vi "Actor Core.vi"(8 "error in (no error)":errorcluster, 11 "MC Screen.lvlib:MC Screen.lvclass":refnum<class "Grid Screen.lvclass">) -> (0 "error out":errorcluster, 3 "Actor out":refnum<class "Actor.lvclass">)   [LabVIEW 2024, in "Grid Screen.lvlib" / "Grid Screen.lvclass"]
uses:
  Grid Screen.lvclass
  <vilib>/ActorFramework/Actor/Actor.lvclass
  <vilib>/Utility/miscctls.llb/LVRectTypeDef.ctl
  Grid Screen.lvclass/Grid Screen.ctl
  <vilib>/ActorFramework/Actor/Actor.lvclass/Actor.ctl
  <vilib>/ActorFramework/Message Enqueuer/Message Enqueuer.lvclass/Message Enqueuer.ctl
  Grid Screen Messages/Button Pressed Msg/Button Pressed Msg.lvclass/Button Pressed Msg.ctl
  <vilib>/ActorFramework/Message Enqueuer/Init from Existing Queue.vi
  <vilib>/ActorFramework/Message Enqueuer/Enqueue.vi
  Grid Screen Messages/Button Pressed Msg/Button Pressed Msg.lvclass
  <vilib>/ActorFramework/Stop Msg/Stop Msg.lvclass
  <vilib>/ActorFramework/Message Priority Queue/Priority Enqueue.vi
  <vilib>/ActorFramework/Message Enqueuer/Message Enqueuer.lvclass
panel:
  out "Cat 1":string="CATEGORY 1"
  out "Cat 2":string="CATEGORY 2"
  out "Cat 3":string="CATEGORY 3"
  out "Cat 4":string="CATEGORY 4"
  out "Cat 5":string="CATEGORY 5"
  out "A1":bool
  out "A2":bool
  out "A3":bool
  out "A4":bool
  out "A5":bool
  out "B1":bool
  out "B2":bool
  out "B3":bool
  out "B4":bool
  out "B5":bool
  out "C1":bool
  out "C2":bool
  out "C3":bool
  out "C4":bool
  out "C5":bool
  out "D1":bool
  out "D2":bool
  out "D3":bool
  out "D4":bool
  out "D5":bool
  out "E1":bool
  out "E2":bool
  out "E3":bool
  out "E4":bool
  out "E5":bool
  in  "Stop":bool
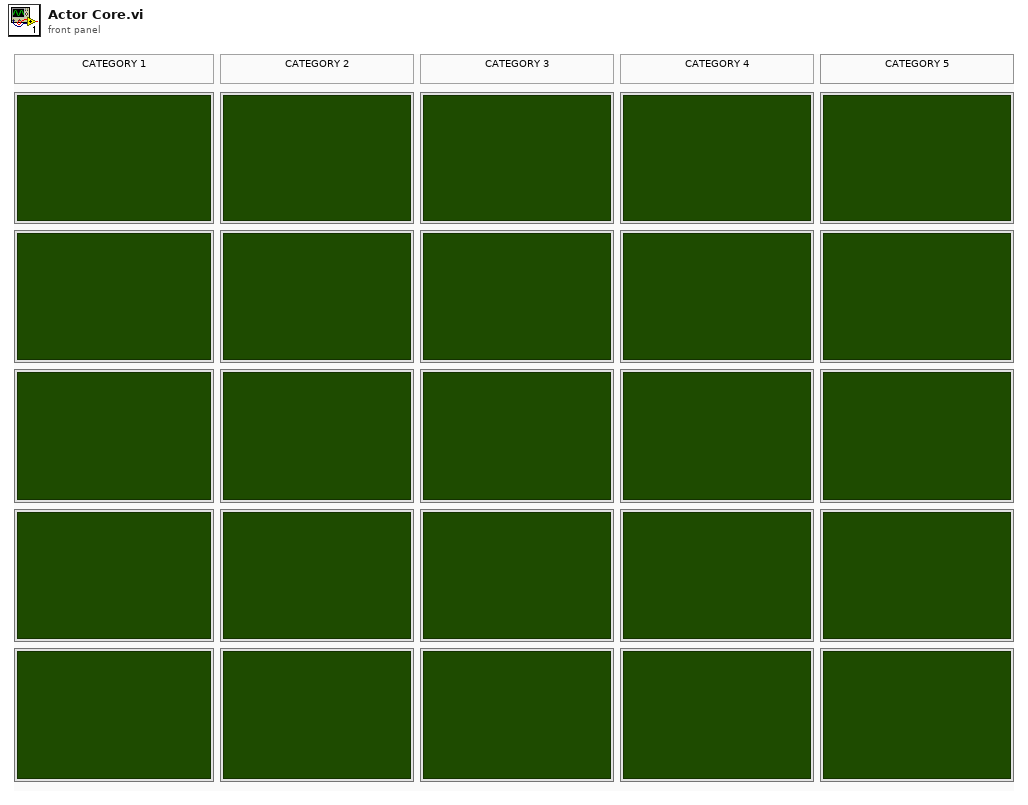
[diagram p1: front panel]
types:
  T1 = enum16{"Sticks Top/Left", "Sticks Bottom/Right", "Proportional"}
  T2 = typedef "LVRectTypeDef.ctl" = cluster{"Left":i16, "Top":i16, "Right":i16, "Bottom":i16}
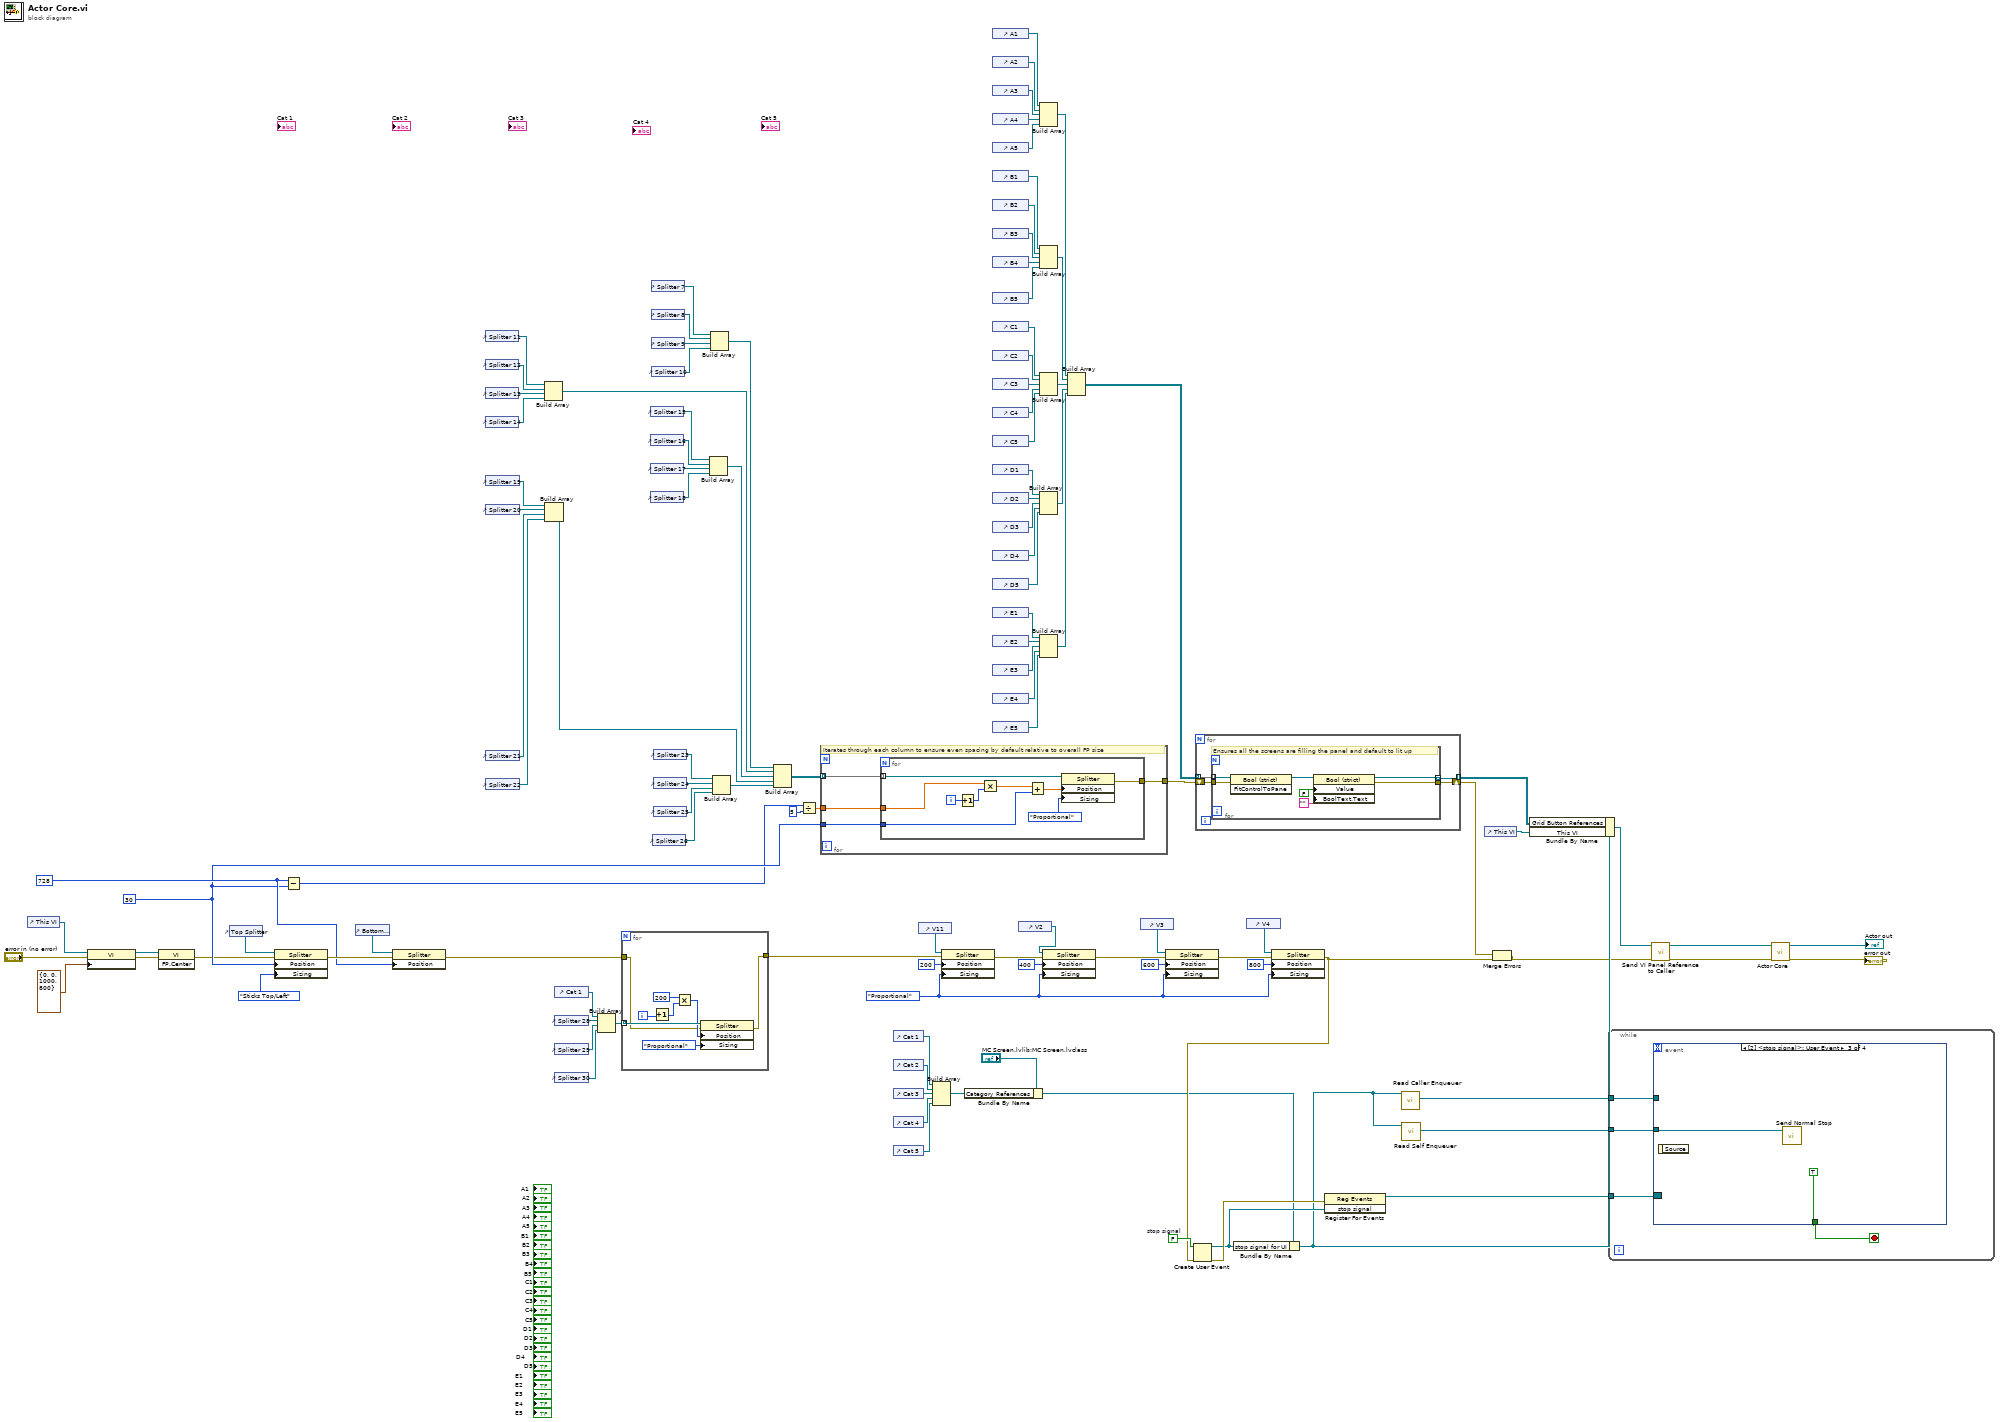
[diagram p0: block diagram]
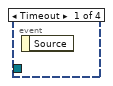
[diagram p2: hidden frame]
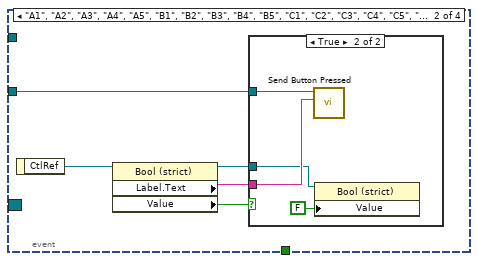
[diagram p3: hidden frame]
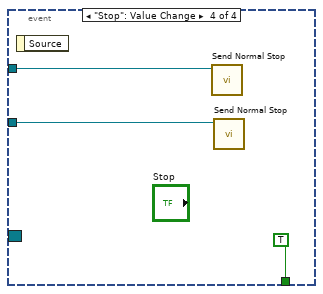
[diagram p5: hidden frame]
diagram:
  w63 = FALSE  # stop signal
  w105 = T1."Proportional" ("Sizing")
  w74 = 728 ("Splitter Position")
  w73 = 30 ("Splitter Position")
  n1 = control-ref of="This VI"() -> (w46:refnum<vi>)
  n2 = property class="VI"(reference=w46, error in="error in (no error)", "Front Panel.WinBounds"=T2 {"Left"=0, "Top"=0, "Right"=1000, "Bottom"=800} ("Front Panel Window:Window Bounds")) -> (reference out=w60:refnum<vi>, error out=w61:errorcluster)
  n3 = invoke class="VI" method="FP.Center"(reference=w60, error in=w61) -> (error out=w54:errorcluster)  [unwired: 1 in, 2 out]
  n4 = control-ref of="Top Splitter"() -> (w116:refnum<vi>)
  n5 = property class="Splitter"(reference=w116, error in=w54, "Position"=w73, "Sizing"=T1."Sticks Top/Left") -> (error out=w114:errorcluster)  [unwired: 1 out]
  n6 = Subtract(x=w74, y=w73) -> (x-y=w72:i32)
  n7 = control-ref of="Bottom Splitter"() -> (w115:refnum<vi>)
  n8 = property class="Splitter"(reference=w115, error in=w114, "Position"=w74) -> (error out=w53:errorcluster)  [unwired: 1 out]
  n9 = control-ref of="Splitter 11"() -> (w96:refnum<vi>)
  n10 = control-ref of="Splitter 12"() -> (w95:refnum<vi>)
  n11 = control-ref of="Splitter 13"() -> (w82:refnum<vi>)
  n12 = control-ref of="Splitter 14"() -> (w81:refnum<vi>)
  n13 = control-ref of="Splitter 19"() -> (w84:refnum<vi>)
  n14 = control-ref of="Splitter 20"() -> (w91:refnum<vi>)
  n15 = control-ref of="Splitter 21"() -> (w90:refnum<vi>)
  n16 = control-ref of="Splitter 22"() -> (w89:refnum<vi>)
  n17 = Build Array(w96, w95, w82, w81) -> (w79:refnum<vi>[])
  n18 = Build Array(w84, w91, w90, w89) -> (w77:refnum<vi>[])
  n19 = control-ref of="Cat 1"() -> (w56:refnum<vi>)
  n20 = control-ref of="Splitter 28"() -> (w57:refnum<vi>)
  n21 = control-ref of="Splitter 29"() -> (w58:refnum<vi>)
  n22 = control-ref of="Splitter 30"() -> (w59:refnum<vi>)
  n23 = Build Array(w56, w57, w58, w59) -> (w55:refnum<vi>[])
  n24 = for {
    tunnel: w55 -> [w125] mode=indexing
    tunnel: [w119] -> w52
    tunnel: w53 -> [w118]
    i -> [w122]
    n25 = Increment(x=w122) -> (x+1=w123:i32)
    n26 = Multiply(x=200, y=w123) -> (x*y=w120:i32)
    n27 = property class="Splitter"(reference=w125, error in=w118, "Position"=w120, "Sizing"=T1."Proportional") -> (error out=w119:errorcluster)  [unwired: 1 out]
  }
  n28 = control-ref of="Splitter 15"() -> (w94:refnum<vi>)
  n29 = control-ref of="Splitter 16"() -> (w83:refnum<vi>)
  n30 = control-ref of="Splitter 17"() -> (w93:refnum<vi>)
  n31 = control-ref of="Splitter 18"() -> (w92:refnum<vi>)
  n32 = control-ref of="Splitter 7"() -> (w100:refnum<vi>)
  n33 = control-ref of="Splitter 8"() -> (w99:refnum<vi>)
  n34 = control-ref of="Splitter 9"() -> (w98:refnum<vi>)
  n35 = control-ref of="Splitter 10"() -> (w97:refnum<vi>)
  n36 = control-ref of="Splitter 26"() -> (w85:refnum<vi>)
  n37 = control-ref of="Splitter 23"() -> (w88:refnum<vi>)
  n38 = control-ref of="Splitter 24"() -> (w87:refnum<vi>)
  n39 = control-ref of="Splitter 25"() -> (w86:refnum<vi>)
  n40 = Build Array(w94, w83, w93, w92) -> (w78:refnum<vi>[])
  n41 = Build Array(w100, w99, w98, w97) -> (w80:refnum<vi>[])
  n42 = Build Array(w88, w87, w86, w85) -> (w76:refnum<vi>[])
  n43 = Build Array(w80, w79, w78, w77, w76) -> (w75:refnum<vi>[][])
  n44 = Divide(x=w72, y=5) -> (x/y=w70:dbl)
  n45 = for {
    tunnel: w75 -> [w129] mode=indexing
    tunnel: [w128] -> w69
    tunnel: w73 -> [w127]
    tunnel: w70 -> [w126]
    # "Iterates through each column to ensure even spacing by default relative to overall FP size"
    n46 = for {
      tunnel: w129 -> [w138] mode=indexing
      tunnel: [w134] -> w128
      tunnel: w127 -> [w131]
      tunnel: w126 -> [w130]
      i -> [w137]
      n47 = Increment(x=w137) -> (x+1=w135:i32)
      n48 = Multiply(x=w130, y=w135) -> (x*y=w133:dbl)
      n49 = Add(x=w133, y=w131) -> (x+y=w132:dbl)
      n50 = property class="Splitter"(reference=w138, "Position"=w132, "Sizing"=T1."Proportional") -> (error out=w134:errorcluster)  [unwired: 1 in, 1 out]
    }
  }
  n51 = control-ref of="Cat 1"() -> (w36:refnum<vi>)
  n52 = control-ref of="Cat 2"() -> (w37:refnum<vi>)
  n53 = control-ref of="Cat 3"() -> (w38:refnum<vi>)
  n54 = control-ref of="Cat 4"() -> (w39:refnum<vi>)
  n55 = control-ref of="Cat 5"() -> (w40:refnum<vi>)
  n56 = control-ref of="V11"() -> (w112:refnum<vi>)
  n57 = Build Array(w36, w37, w38, w39, w40) -> (w33:refnum<vi>[])
  n58 = property class="Splitter"(reference=w112, error in=w52, "Position"=200 ("Splitter Position"), "Sizing"=w105) -> (error out=w103:errorcluster)  [unwired: 1 out]
  n59 = Bundle By Name(cluster="MC Screen.lvlib:MC Screen.lvclass", "Category References"=w33) -> (w34:refnum<class "Grid Screen.lvclass">)
  n60 = control-ref of="A1"() -> (w32:refnum<vi>)
  n61 = control-ref of="A2"() -> (w31:refnum<vi>)
  n62 = control-ref of="A3"() -> (w30:refnum<vi>)
  n63 = control-ref of="A4"() -> (w29:refnum<vi>)
  n64 = control-ref of="A5"() -> (w28:refnum<vi>)
  n65 = control-ref of="B1"() -> (w27:refnum<vi>)
  n66 = control-ref of="B2"() -> (w26:refnum<vi>)
  n67 = control-ref of="B3"() -> (w25:refnum<vi>)
  n68 = control-ref of="B4"() -> (w24:refnum<vi>)
  n69 = control-ref of="B5"() -> (w23:refnum<vi>)
  n70 = control-ref of="C1"() -> (w22:refnum<vi>)
  n71 = control-ref of="C2"() -> (w21:refnum<vi>)
  n72 = control-ref of="C3"() -> (w20:refnum<vi>)
  n73 = control-ref of="C4"() -> (w19:refnum<vi>)
  n74 = control-ref of="C5"() -> (w18:refnum<vi>)
  n75 = control-ref of="D1"() -> (w17:refnum<vi>)
  n76 = control-ref of="D2"() -> (w16:refnum<vi>)
  n77 = control-ref of="D3"() -> (w15:refnum<vi>)
  n78 = control-ref of="D4"() -> (w14:refnum<vi>)
  n79 = control-ref of="D5"() -> (w13:refnum<vi>)
  n80 = control-ref of="E1"() -> (w12:refnum<vi>)
  n81 = control-ref of="E2"() -> (w11:refnum<vi>)
  n82 = control-ref of="E3"() -> (w10:refnum<vi>)
  n83 = control-ref of="E4"() -> (w9:refnum<vi>)
  n84 = control-ref of="E5"() -> (w8:refnum<vi>)
  n85 = control-ref of="V2"() -> (w110:refnum<vi>)
  n86 = Build Array(w32, w31, w30, w29, w28) -> (w7:refnum<vi>[])
  n87 = Build Array(w27, w26, w25, w24, w23) -> (w6:refnum<vi>[])
  n88 = Build Array(w22, w21, w20, w19, w18) -> (w5:refnum<vi>[])
  n89 = Build Array(w17, w16, w15, w14, w13) -> (w4:refnum<vi>[])
  n90 = Build Array(w12, w11, w10, w9, w8) -> (w3:refnum<vi>[])
  n91 = property class="Splitter"(reference=w110, error in=w103, "Position"=400 ("Splitter Position"), "Sizing"=w105) -> (error out=w102:errorcluster)  [unwired: 1 out]
  n92 = Build Array(w7, w6, w5, w4, w3) -> (w2:refnum<vi>[][])
  n93 = control-ref of="V3"() -> (w108:refnum<vi>)
  n94 = property class="Splitter"(reference=w108, error in=w102, "Position"=600 ("Splitter Position"), "Sizing"=w105) -> (error out=w101:errorcluster)  [unwired: 1 out]
  n95 = for {
    shift-right: [w141] -> w44
    shift-left: w69 -> [w142]
    tunnel: w2 -> [w140] mode=indexing
    tunnel: [w139] -> w1 mode=indexing
    n96 = for {
      tunnel: w140 -> [w145] mode=indexing
      tunnel: w142 -> [w149]
      tunnel: [w146] -> w141
      tunnel: [w144] -> w139 mode=indexing
      # "Ensures all the screens are filling the panel and default to lit up"
      n97 = invoke class="Bool (strict)" method="FitControlToPane"(reference=w145, error in=w149) -> (reference out=w148:refnum<vi>)  [unwired: 1 in, 2 out]
      n98 = property class="Bool (strict)"(reference=w148, "Value"=FALSE, "BoolText.Text"="" ("Boolean Text.Text")) -> (reference out=w144:refnum<vi>, error out=w146:errorcluster)  [unwired: 1 in]
    }
  }
  n99 = control-ref of="V4"() -> (w106:refnum<vi>)
  n100 = property class="Splitter"(reference=w106, error in=w101, "Position"=800 ("Splitter Position"), "Sizing"=w105) -> (error out=w43:errorcluster)  [unwired: 1 out]
  n101 = Create User Event(user event datatype=w63, error in=w43) -> (user event=w65:refnum<user-event>, error out=w66:errorcluster)
  n102 = Bundle By Name(cluster=w34, "stop signal for UI"=w65) -> (w51:refnum<class "Grid Screen.lvclass">)
  n103 = register-events(error in=w66, w65) -> (reference out=w64:refnum<event-registration>)  [unwired: 1 in, 1 out]
  n104 = call <vilib>:"Read Caller Enqueuer.vi"("Actor"=w51) -> ("Caller Enqueuer"=w48:refnum<class "Message Enqueuer.lvclass">)  [unwired: 10 in]
  n105 = call <vilib>:"Read Self Enqueuer.vi"("Actor"=w51) -> ("Self Enqueuer"=w62:refnum<class "Message Enqueuer.lvclass">)  [unwired: 10 in]
  n106 = control-ref of="This VI"() -> (w47:refnum<vi>)
  n107 = Merge Errors(w44, w43) -> (w42:errorcluster)
  n108 = Bundle By Name(cluster=w51, "Grid Button References"=w1, "This VI"=w47) -> (w50:refnum<class "Grid Screen.lvclass">)
  n109 = while {
    tunnel: w48 -> [w152]
    tunnel: w64 -> [w151]
    tunnel: w62 -> [w150]
    stop <- w153 stop-if-true
    n110 = event shown="[2] <stop signal>: User Event" {
      selector: w151 -> [_ _ _ _]
      dyn-events: _ -> [_ _ _ _]
      timeout: _ -> [_ _ _ _]
      tunnel: [_ _ TRUE TRUE] -> w153
      tunnel: w152 -> [_ _ _ w165]
      tunnel: w150 -> [_ w157 w163 w166]
      event Timeout {
        n111 = event-data() -> ()  [unwired: 1 in, 1 out]
      }
      event "A1", "A2", "A3", "A4", "A5", "B1", "B2", "B3", "B4", "B5", "C1", "C2", "C3", "C4", "C5", "D1", "D2", "D3", "D4", "D5", "E1", "E2", "E3", "E4", "E5": Mouse Down {
        n112 = event-data() -> ("CtlRef"=w158:refnum<vi>)  [unwired: 1 in]
        n113 = property class="Bool (strict)"(reference=w158) -> (reference out=w154:refnum<vi>, "Label.Text"=w156:string, "Value"=w155:bool)  [unwired: 1 in, 1 out]
        n114 = case shown="True" w155 {
          tunnel: w157 -> [_ w162]
          tunnel: w156 -> [_ w161]
          tunnel: w154 -> [_ w159]
          frame False {
          }
          frame True {
            n115 = call "Send Button Pressed.vi"("Button Text"=w161, "Message Enqueuer"=w162) -> ()  [unwired: 8 in, 2 out]
            n116 = property class="Bool (strict)"(reference=w159, "Value"=FALSE) -> ()  [unwired: 1 in, 2 out]
          }
        }
      }
      event User Event {
        n117 = event-data() -> ()  [unwired: 1 in, 1 out]
        n118 = call <vilib>:"Send Normal Stop.vi"("Message Enqueuer"=w163) -> ()  [unwired: 10 in, 1 out]
      }
      event "Stop": Value Change {
        n119 = event-data() -> ()  [unwired: 1 in, 1 out]
        n120 = call <vilib>:"Send Normal Stop.vi"("Message Enqueuer"=w165) -> ()  [unwired: 10 in, 1 out]
        n121 = call <vilib>:"Send Normal Stop.vi"("Message Enqueuer"=w166) -> ()  [unwired: 10 in, 1 out]
      }
    }
  }
  n122 = call "Send VI Panel Reference to Caller.vi"("error in (no error)"=w42, "Grid Screen in"=w50) -> ("error out"=w41:errorcluster, "Grid Screen out"=w49:refnum<class "Grid Screen.lvclass">)  [unwired: 8 in]
  n123 = call-parent "Actor Core.vi"("error in"=w41, "Actor in"=w49) -> ("error out"=→"error out":errorcluster, "Actor out"=→"Actor out":refnum<class "Actor.lvclass">)  [unwired: 8 in]
